vi "stop.vi"(8 "error in (no error)":errorcluster, 11 "TestSeries in":refnum<class "TestSeries.lvclass">) -> (0 "error out":errorcluster, 3 "TestSeries out":refnum<class "TestSeries.lvclass">)   [LabVIEW 2015, in "TestSeries.lvclass"]
uses:
  TestSeries.lvclass
  TestSeries.lvclass/TestSeries.ctl
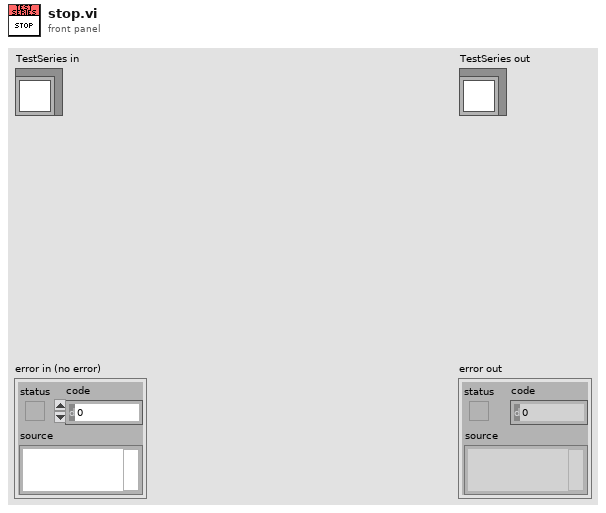
[diagram p1: front panel]
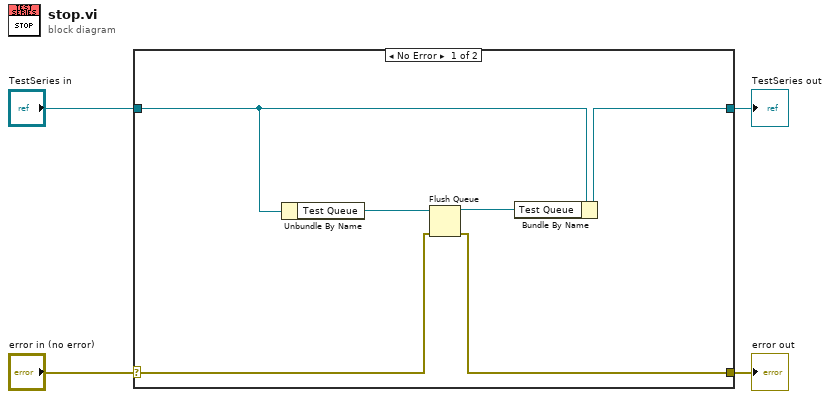
[diagram p0: block diagram]
diagram:
  n1 = case shown="No Error" "error in (no error)" {
    selector: "error in (no error)" -> [w5 w12]
    tunnel: [w6 w12] -> w3
    tunnel: [w8 w11] -> w1
    tunnel: "TestSeries in" -> [w9 w11]
    frame No Error {
      n2 = Unbundle By Name(w9) -> ("Test Queue"=w10:refnum<queue>)
      n3 = Flush Queue(queue=w10, error in (no error)=w5) -> (queue out=w7:refnum<queue>, error out=w6:errorcluster)  [unwired: 1 out]
      n4 = Bundle By Name(cluster=w9, "Test Queue"=w7) -> (w8:refnum<class "TestSeries.lvclass">)
    }
    frame Error {
    }
  }
  "error out" <- w3
  "TestSeries out" <- w1
